vi "wait for temp to settle.vi"(5 "Current setpoint":dbl format="%.2f", 7 "Timing Control Parameters In":T1={"N cycles for averaging"=30, "N points per measurement"=1000, "Measurment time interval"=2e-05} {"Measurment time interval" format="%.2e"}, 11 "error in":errorcluster) -> (8 "Timing Control Parameters Out":T1={"N cycles for averaging"=30, "N points per measurement"=1000, "Measurment time interval"=2e-05} {"Measurment time interval" format="%.2e"}, 15 "error out":errorcluster)   [LabVIEW 2016]
doc: "This subvi gives the setpoint for the current stage of the experiment to the global controls of the temperature control subvi, and waits for the subvi to cause the bug to reach the setpoint\n\nPaul K Dixon\nPhysics 350\nCSUSB Physics"
uses:
  temp control/globals/temp control global variables.vi
  globals/C(T) global variables.vi
panel:
  out "time in this wait cycle (sec)":dbl format="%.1f"
  in  "Proceed":bool
  # "C(T) Waiting for Temp to settle"
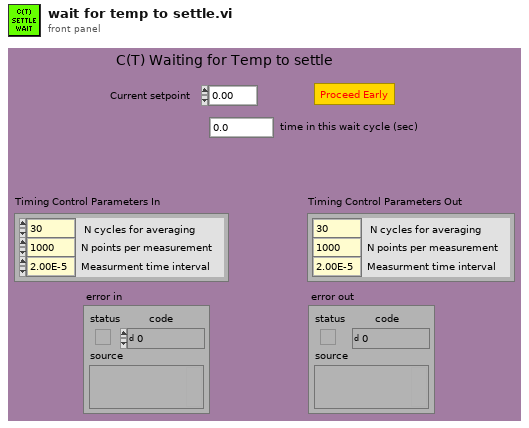
[diagram p1: front panel]
types:
  T1 = cluster{"N cycles for averaging":i32, "N points per measurement":i32, "Measurment time interval":dbl}
  T2 = typedef "control parameters.ctl" = cluster{"Setpoint":dbl, "Control bandwidth":dbl, "Settle bandwidth":dbl, "Integral time":dbl, "Int\non":bool, "Derivative time":dbl, "Der\non":bool, "Settle time":dbl}
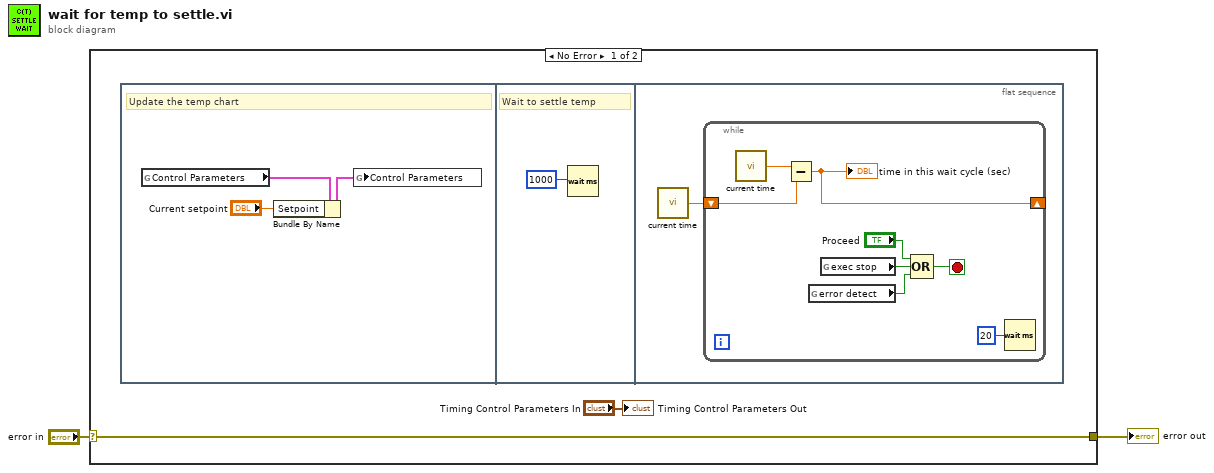
[diagram p0: block diagram]
diagram:
  n1 = case shown="No Error" "error in" {
    selector: "error in" -> [w3 w18]
    tunnel: [w3 w18] -> w1
    frame No Error {
      n2 = flat-sequence {
        frame #0 {
          # "Update the temp chart"
          n3 = global read "temp control global variables.vi" "Control Parameters"() -> (w7:T2)
          n4 = Bundle By Name(cluster=w7, "Setpoint"="Current setpoint") -> (w5:T2)
          n5 = global write "temp control global variables.vi" "Control Parameters"(w5) -> ()
        }
        frame #1 {
          # "Wait to settle temp"
          n6 = Wait (ms)(milliseconds to wait=u32 1000) -> ()  [unwired: 1 out]
        }
        frame #2 {
          n7 = call "current time.vi"() -> ("current time (sec)"=w9:dbl)
          n8 = while {
            shift-right: [w15] -> _
            shift-left: w9 -> [w16]
            stop <- w10 stop-if-true
            n9 = call "current time.vi"() -> ("current time (sec)"=w17:dbl)
            n10 = Subtract(x=w17, y=w16) -> (x-y=w15:dbl)
            "time in this wait cycle (sec)" <- w15
            n11 = global read "C(T) global variables.vi" "error detect"() -> (w11:bool)
            n12 = global read "C(T) global variables.vi" "exec stop"() -> (w12:bool)
            n13 = Compound Arithmetic op=OR("Proceed", w12, w11) -> (w10:bool)
            n14 = Wait (ms)(milliseconds to wait=u32 20) -> ()  [unwired: 1 out]
          }
        }
      }
      "Timing Control Parameters Out" <- "Timing Control Parameters In"
    }
    frame Error {
    }
  }
  "error out" <- w1
